vi "Config.vi"(8 "error in (no error)":errorcluster, 10 "Setting":T1={"Resolution (Digits)"=5.5, "Current Source (Amps)"=0.001, "Range"=2.0, "Measurement Type"=enum."DC Volts"} {"Range" format="%.2p"; "Current Source (Amps)" items=["1uA"=1e-06, "10uA"=1e-05, "100uA"=0.0001, "1mA"=0.001]; "Resolution (Digits)" items=["3 1/2"=3.5, "4 1/2"=4.5, "5 1/2"=5.5, "6 1/2"=6.5, "7 1/2"=7.5]}, 11 "NI DMM4072 in":refnum<class "NI DMM4072.lvclass">) -> (0 "error out":errorcluster, 3 "NI DMM4072 out":refnum<class "NI DMM4072.lvclass">)   [LabVIEW 2021, in "Concrete.lvlib" / "NI DMM4072.lvclass"]
uses:
  NI DMM4072.lvclass
  NI DMM4072.lvclass/NI DMM4072.ctl
  <instrlib>/niDMM/nidmm.llb/niDMM Configure Measurement Digits.vi
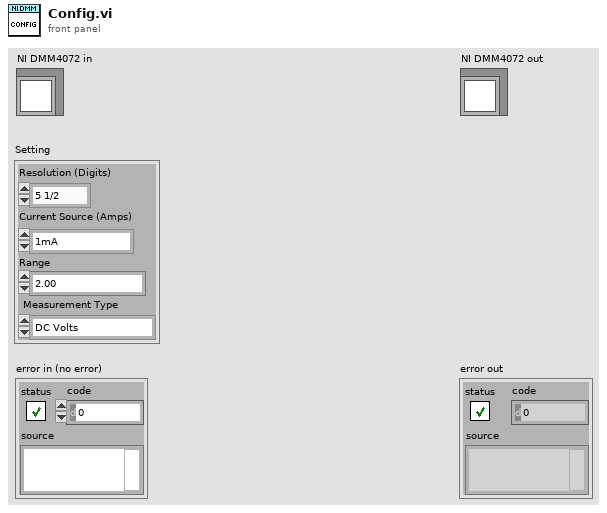
[diagram p1: front panel]
types:
  T1 = cluster{"Resolution (Digits)":dbl, "Current Source (Amps)":dbl, "Range":dbl, "Measurement Type":enum16{"DC Volts", "AC Volts", "DC Current", "AC Current", "2-wire Resistance", "4-wire Resistance", "Diode", "Frequency", "Period", "AC Volts DC Coupled", "Capacitance", "Inductance", "Temperature"}}
  T2 = enum16{"DC Volts", "AC Volts", "DC Current", "AC Current", "2-wire Resistance", "4-wire Resistance", "Diode", "Frequency", "Period", "AC Volts DC Coupled", "Capacitance", "Inductance", "Temperature"}
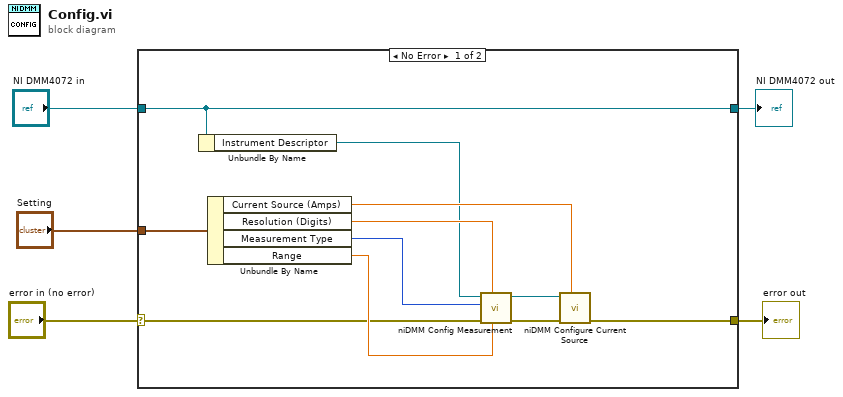
[diagram p0: block diagram]
diagram:
  n1 = case shown="No Error" "error in (no error)" {
    selector: "error in (no error)" -> [w10 w18]
    tunnel: [w9 w18] -> w4
    tunnel: [w7 w17] -> w2
    tunnel: "NI DMM4072 in" -> [w7 w17]
    tunnel: "Setting" -> [w8 _]
    frame No Error {
      n2 = Unbundle By Name(w7) -> ("Instrument Descriptor"=w6:refnum<k15>)
      n3 = Unbundle By Name(w8) -> ("Current Source (Amps)"=w16:dbl, "Resolution (Digits)"=w13:dbl, "Measurement Type"=w14:T2, "Range"=w15:dbl)
      n4 = call-poly <instrlib>:"niDMM Config Measurement.vi"("Range"=w15, "Resolution in Digits"=w13, "error in (no error)"=w10, "Function"=w14, "instrument handle"=w6) -> ("error out"=w11:errorcluster, "instrument handle out"=w12:refnum<k15>)  [unwired: 5 out]
      n5 = call <instrlib>:"niDMM Configure Current Source.vi"("Current Source"=w16, "error in (no error)"=w11, "instrument handle"=w12) -> ("error out"=w9:errorcluster)  [unwired: 1 in, 7 out]
    }
    frame Error {
    }
  }
  "error out" <- w4
  "NI DMM4072 out" <- w2
